vi "Refill.vi"(0 "object in":refnum<class "CetoniPump.lvclass">, 5 "error in (no error)":errorcluster) -> (14 "object out":refnum<class "CetoniPump.lvclass">, 19 "error out":errorcluster)   [LabVIEW 2024, in "CetoniPump.lvclass"]
uses:
  CetoniPump.lvclass
  CetoniPump.lvclass/CetoniPump.ctl
  Users/Lab user/AppData/Local/CETONI_SDK/lib/labview/labbCAN_Pump_API/labbCAN_Pump_API.lvlib
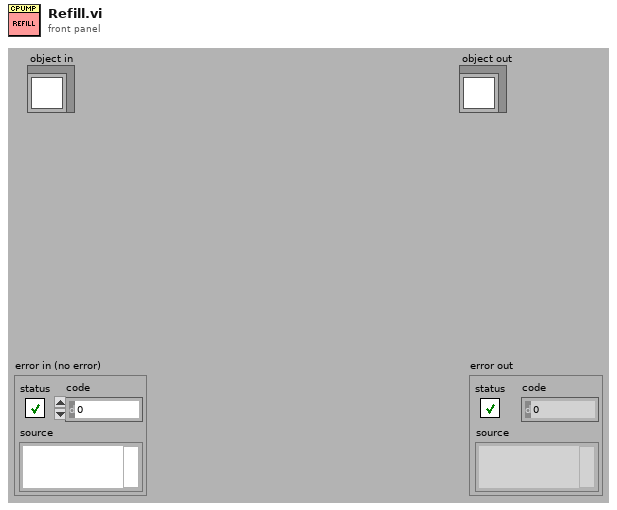
[diagram p1: front panel]
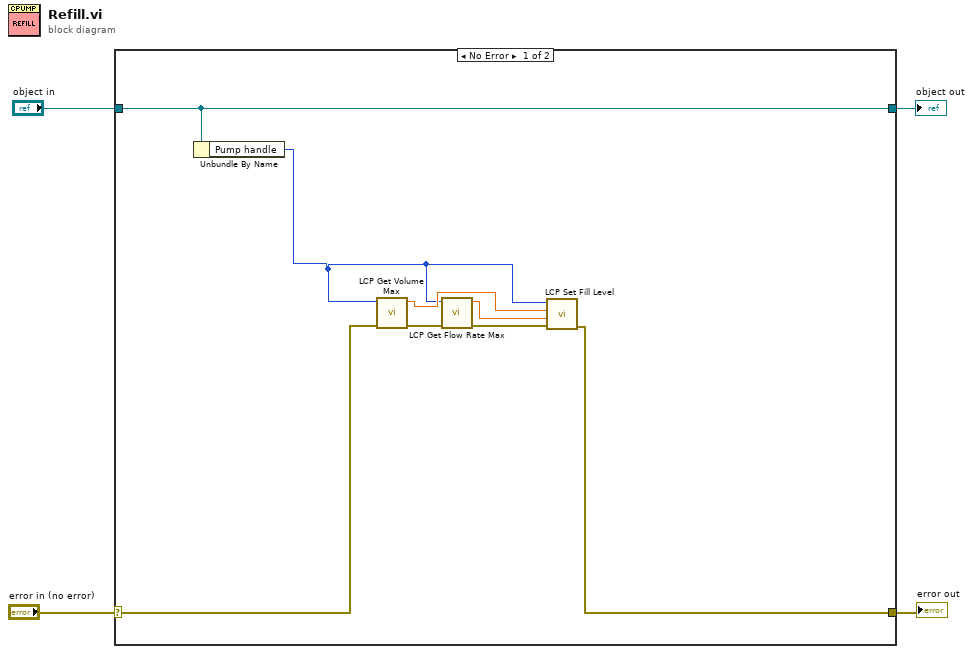
[diagram p0: block diagram]
diagram:
  n1 = case shown="No Error" "error in (no error)" {
    selector: "error in (no error)" -> [w6 w14]
    tunnel: [w5 w14] -> w3
    tunnel: [w12 w13] -> w1
    tunnel: "object in" -> [w12 w13]
    frame No Error {
      n2 = Unbundle By Name(w12) -> ("Pump handle"=w7:i64)
      n3 = call "LCP Get Volume Max.vi"("error in (no error)"=w6, "Pump Handle"=w7) -> ("error out"=w11:errorcluster, "Maximum Volume"=w8:dbl)  [unwired: 8 in]
      n4 = call "LCP Get Flow Rate Max.vi"("error in (no error)"=w11, "Pump Handle"=w7) -> ("error out"=w10:errorcluster, "Maximum Flow Rate"=w9:dbl)  [unwired: 8 in]
      n5 = call "LCP Set Fill Level.vi"("error in (no error)"=w10, "Flow"=w9, "Level"=w8, "Pump Handle"=w7) -> ("error out"=w5:errorcluster)  [unwired: 7 in]
    }
    frame Error {
    }
  }
  "error out" <- w3
  "object out" <- w1
